vi "rqcAlice Cascade sync ui (Low Level Example).vi"() -> ()   [LabVIEW 2019]
panel:
  in  "picture path":path=path "../python_scripts/cascade_alice.py"
  out "cascade executed":bool=TRUE
  in  "local Corrected Alice's key path":path
  out "picture sent":bool=TRUE
  in  "send Bob the picture":bool
  in  "QBER":dbl
  in  "local Raw Alice's key path":path=path "../python_scripts/cascade_alice.py"
  out "picture demo script path":path=path "../python_scripts/cascade_alice.py"
  in  "error in":errorcluster
  in  "cascade switch":bool
  in  "stop":bool
  in  "Bob's port":string
  in  "Bob's IP":string
  out "?":T1
  out "?":picture
  out "cascade script path":path=path "../python_scripts/cascade_alice.py"
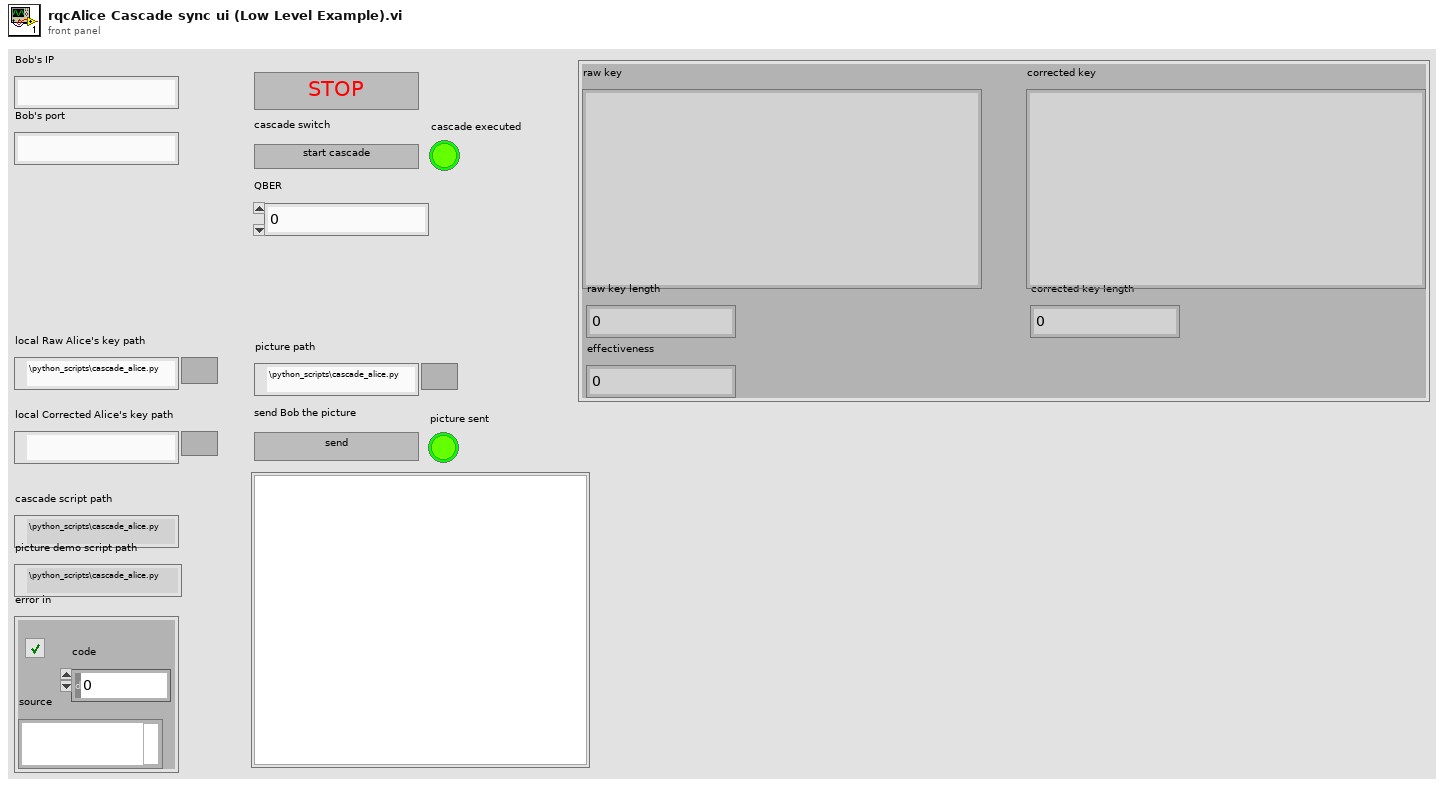
[diagram p1: front panel]
types:
  T1 = cluster{"raw key length":i32, "corrected key":string, "corrected key length":i32, "effectiveness":dbl, "raw key":string}
  T2 = typedef "imagedata.ctl" = cluster{"image type":i32, "image depth":i32, "image":u8[], "mask":u8[], "colors":u32[], "Rectangle":cluster{"left":i16, "top":i16, "right":i16, "bottom":i16}}
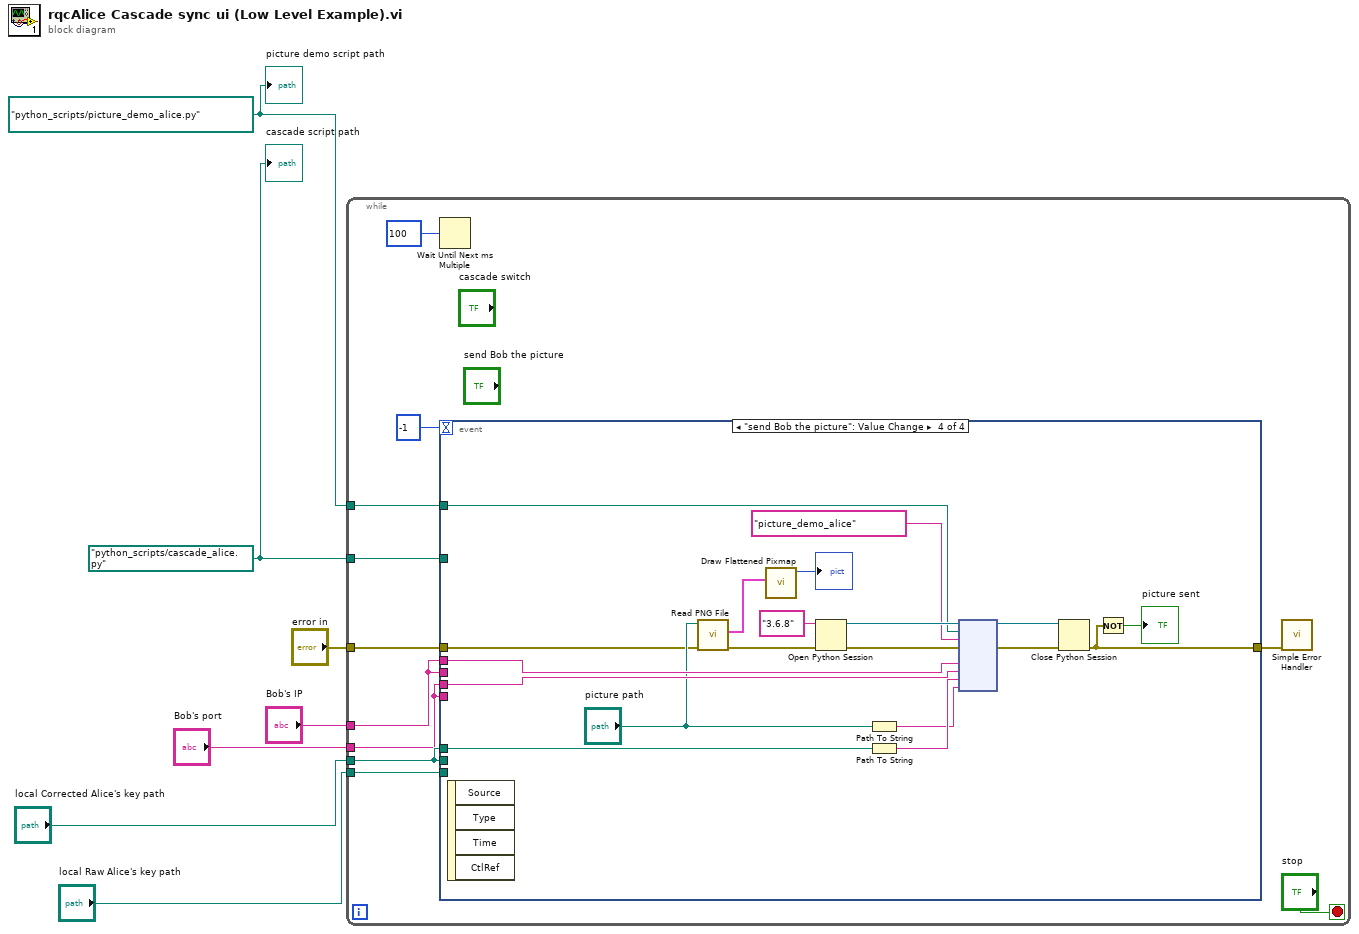
[diagram p0: block diagram]
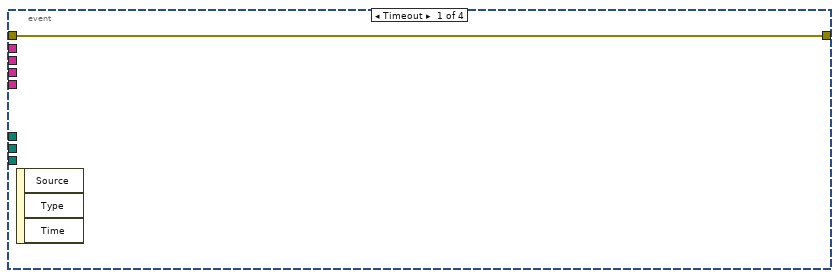
[diagram p2: hidden frame]
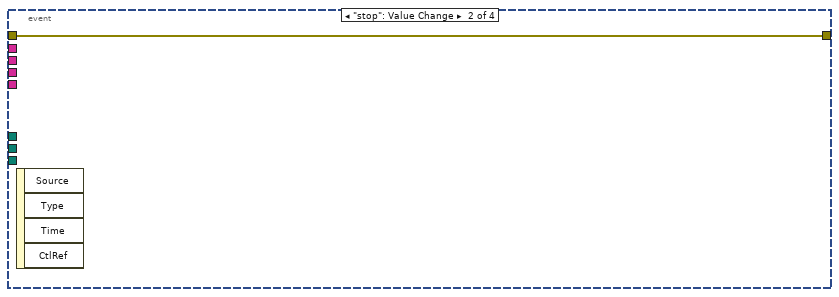
[diagram p3: hidden frame]
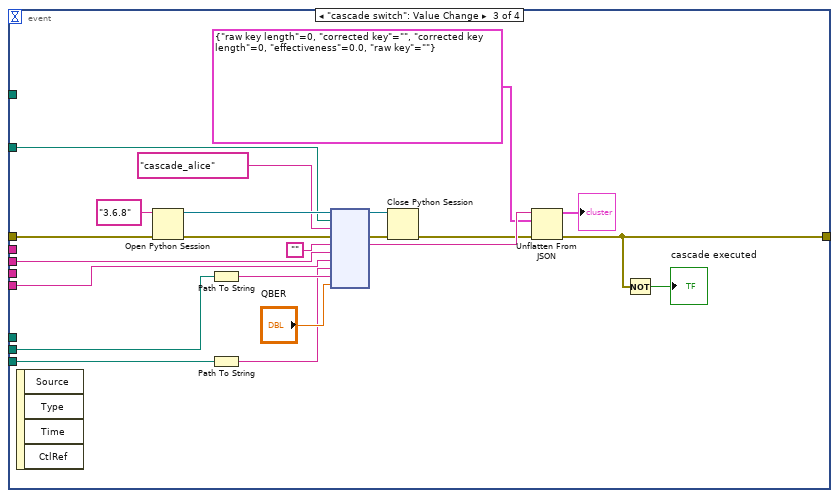
[diagram p4: hidden frame]
diagram:
  w3 = path "python_scripts/picture_demo_alice.py" ("module path")
  w4 = path "python_scripts/cascade_alice.py"
  n1 = while {
    tunnel: "error in" -> [w15]
    tunnel: "Bob's port" -> [w10]
    tunnel: "Bob's IP" -> [w11]
    tunnel: w4 -> [w17]
    tunnel: w3 -> [w12]
    tunnel: "local Raw Alice's key path" -> [w14]
    tunnel: "local Corrected Alice's key path" -> [w13]
    stop <- "stop" stop-if-true
    n2 = Wait Until Next ms Multiple(millisecond multiple=u32 100) -> ()  [unwired: 1 out]
    n3 = event shown="[3] \"send Bob the picture\": Value Change" {
      selector: _ -> [_ _ _ _]
      dyn-events: _ -> [_ _ _ _]
      timeout: -1 -> [_ _ _ _]
      tunnel: w13 -> [_ _ w32 _]
      tunnel: w14 -> [_ _ w31 _]
      tunnel: w17 -> [_ _ w28 _]
      tunnel: w11 -> [_ _ w25 _]
      tunnel: w10 -> [_ _ w24 _]
      tunnel: w15 -> [w19 w20 w22 w45]
      tunnel: w13 -> [_ _ _ w54]
      tunnel: w12 -> [_ _ _ w52]
      tunnel: w11 -> [_ _ _ w50]
      tunnel: w10 -> [_ _ _ w49]
      tunnel: [w19 w20 w21 w43] -> w9
      event Timeout {
        n4 = event-data() -> ()  [unwired: 1 in, 3 out]
      }
      event "stop": Value Change {
        n5 = event-data() -> ()  [unwired: 1 in, 4 out]
      }
      event "cascade switch": Value Change {
        n6 = event-data() -> ()  [unwired: 1 in, 4 out]
        n7 = Open Python Session(python version="3.6.8" ("Python version"), 3:w22) -> (session out=w33:refnum<k35>, error out=w34:errorcluster)  [unwired: 1 in]
        n8 = Path To String(path=w32) -> (string=w39:string)
        n9 = Path To String(path=w31) -> (string=w37:string)
        n10 = node(w33, w28, "cascade_alice" ("function name"), w34, "", w25, w24, w37, w39, "QBER") -> (w35:refnum<k35>, w36:errorcluster, w41:string)  [unwired: 5 in, 2 out]
        n11 = Close Python Session(session in=w35, error in=w36) -> (11:w40:errorcluster)
        n12 = Unflatten From JSON(JSON string=w41, type and defaults=T1 {"raw key length"=0, "corrected key"="", "corrected key length"=0, "effectiveness"=0.0, "raw key"=""}, error in (no error)=w40) -> (value=→"?":T1, error out=w21:errorcluster)  [unwired: 4 in]
        n13 = Not(x=w21) -> (.not. x?=→"cascade executed":bool)
      }
      event "send Bob the picture": Value Change {
        n14 = event-data() -> ()  [unwired: 1 in, 4 out]
        n15 = call <vilib>:"Read PNG File.vi"("error in (no error)"=w45, "path to PNG file"="picture path") -> ("error out"=w46:errorcluster, "image data"=w47:T2)  [unwired: 7 in, 1 out]
        n16 = call <vilib>:"Draw Flattened Pixmap.vi"("image data"=w47) -> ("new picture"=→"?":picture)  [unwired: 8 in]
        n17 = Open Python Session(python version="3.6.8" ("Python version"), 3:w46) -> (session out=w57:refnum<k35>, error out=w58:errorcluster)  [unwired: 1 in]
        n18 = Path To String(path="picture path") -> (string=w44:string)
        n19 = Path To String(path=w54) -> (string=w61:string)
        n20 = node(w57, w52, "picture_demo_alice" ("function name"), w58, w50, w49, w61, w44) -> (w59:refnum<k35>, w60:errorcluster)  [unwired: 6 in, 2 out]
        n21 = Close Python Session(session in=w59, error in=w60) -> (11:w43:errorcluster)
        n22 = Not(x=w43) -> (.not. x?=→"picture sent":bool)
      }
    }
    n23 = call <vilib>:"Simple Error Handler.vi"("error in (no error)"=w9) -> ()  [unwired: 4 in, 5 out]
  }
  "cascade script path" <- w4
  "picture demo script path" <- w3
